vi "Get Dist From Two Points.vi"(8 "error in (no error)":errorcluster caption="错误输入（无错误）", 10 "Point 输入":refnum<class "Point.lvclass"> caption="DNL_LabVIEW Object in", 11 "Point 输入":refnum<class "Point.lvclass"> caption="DNL_LabVIEW Object in") -> (0 "error out":errorcluster caption="错误输出", 2 "Dist":dbl, 3 "Point 输出":refnum<class "Point.lvclass"> caption="DNL_LabVIEW Object out")   [LabVIEW 2011, in "Point.lvclass"]
uses:
  Point.lvclass
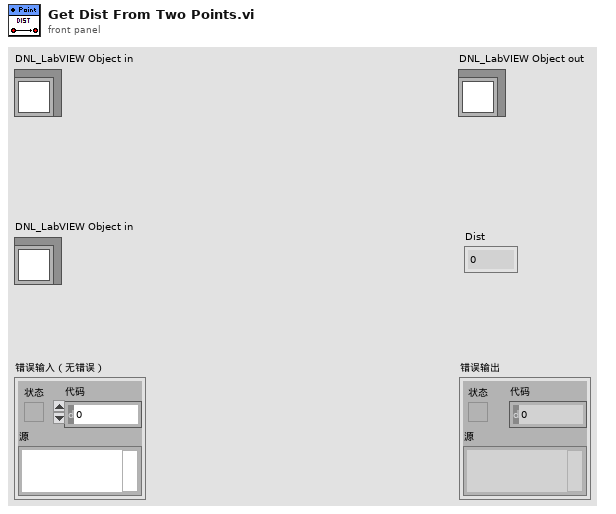
[diagram p1: front panel]
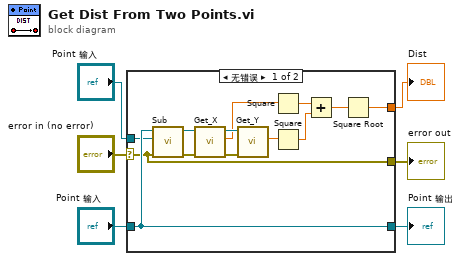
[diagram p0: block diagram]
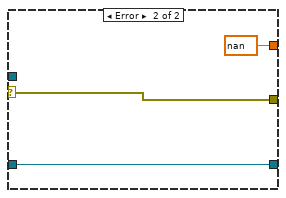
[diagram p2: hidden frame]
diagram:
  n1 = case shown="无错误" "error in (no error)" {
    selector: "error in (no error)" -> [w15 w22]
    tunnel: [w15 w22] -> w5
    tunnel: [w19 w21] -> w3
    tunnel: "Point 输入" -> [w19 w21]
    tunnel: "Point 输入" -> [w18 _]
    tunnel: [w7 nan] -> w1
    frame No Error {
      n2 = call "Sub.vi"("error in (no error)"=w15, 10:"Point 输入"=w18, 11:"Point 输入"=w19) -> ("error out"=w16:errorcluster, "Point 输出"=w17:refnum<class "Point.lvclass">)  [unwired: 7 in]
      n3 = call "Get_X.vi"("error in (no error)"=w16, "Point输入"=w17) -> ("error out"=w13:errorcluster, "X"=w12:dbl, "Point输出"=w14:refnum<class "Point.lvclass">)  [unwired: 7 in]
      n4 = call "Get_Y.vi"("error in (no error)"=w13, "Point输入"=w14) -> ("Y"=w11:dbl)  [unwired: 7 in, 2 out]
      n5 = Square(x=w12) -> (x^2=w10:dbl)
      n6 = Square(x=w11) -> (x^2=w9:dbl)
      n7 = Add(x=w10, y=w9) -> (x+y=w8:dbl)
      n8 = Square Root(x=w8) -> (sqrt(x)=w7:dbl)
    }
    frame Error {
    }
  }
  "error out" <- w5
  "Point 输出" <- w3
  "Dist" <- w1
